vi "ToggleIndicator.vi"(11 "cSonicShifter":bool) -> (3 "Actuate?":bool)   [LabVIEW 2013]
uses:
  ToggleStates.ctl
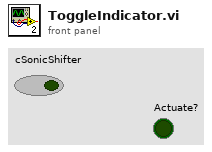
[diagram p1: front panel]
types:
  T1 = typedef "ToggleStates.ctl" = enum16{"Retract2", "Actuate1", "Actuate2", "Retract1"}
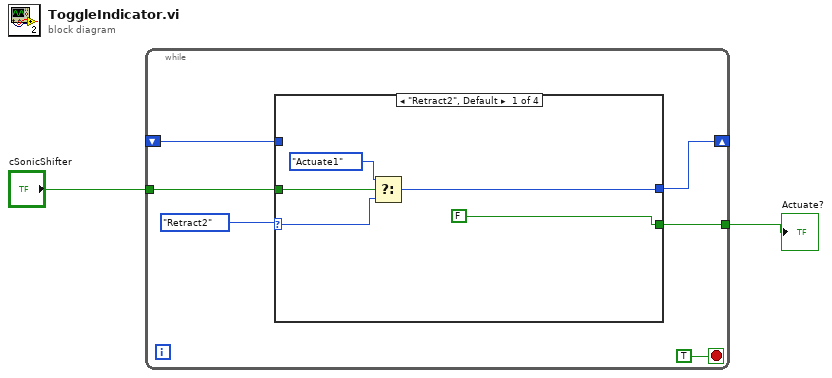
[diagram p0: block diagram]
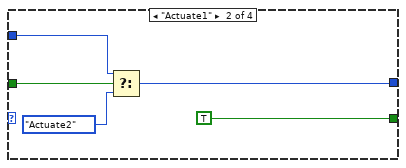
[diagram p2: hidden frame]
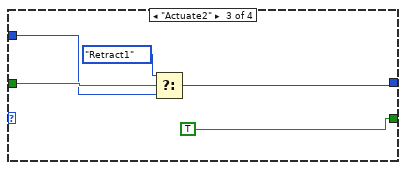
[diagram p3: hidden frame]
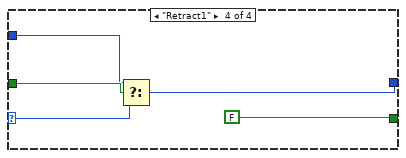
[diagram p4: hidden frame]
diagram:
  n1 = while {
    tunnel: "cSonicShifter" -> [w6]
    shift-right: [w5] -> _
    shift-left: _ -> [w4]
    tunnel: [w3] -> w1
    stop <- TRUE stop-if-true
    n2 = case shown="\"Retract2\", Default" ToggleStates."Retract2" ("Enum") {
      selector: ToggleStates."Retract2" ("Enum") -> [w12 _ _ w24]
      tunnel: w6 -> [w13 w18 w23 w27]
      tunnel: [w10 w16 w19 w25] -> w5
      tunnel: w4 -> [_ w15 w21 w26]
      tunnel: [FALSE TRUE TRUE FALSE] -> w3
      frame "Retract2", Default {
        n3 = Select(t=ToggleStates."Actuate1" ("Enum"), s=w13, f=w12) -> (s? t:f=w10:T1)
      }
      frame "Actuate1" {
        n4 = Select(t=w15, s=w18, f=ToggleStates."Actuate2" ("Enum")) -> (s? t:f=w16:T1)
      }
      frame "Actuate2" {
        n5 = Select(t=ToggleStates."Retract1" ("Enum"), s=w23, f=w21) -> (s? t:f=w19:T1)
      }
      frame "Retract1" {
        n6 = Select(t=w26, s=w27, f=w24) -> (s? t:f=w25:T1)
      }
    }
  }
  "Actuate?" <- w1
